vi "Set Master Info.vi"(8 "error in (no error)":errorcluster, 9 "Master #":u32, 10 "Master Name":string, 11 "Item Ref in":T1 format="%.0x") -> (0 "error out":errorcluster, 3 "Item Ref out":T1 format="%.0x")   [LabVIEW 2016, in "Scan Engine Custom Device.lvlib"]
uses:
  Scan Engine Custom Device.lvlib
  <vilib>/NI Veristand/Custom Device API/Custom Device Item Ref.ctl
  Globals/Property Strings.vi
  <vilib>/NI Veristand/Custom Device API/Set Item Property (U32).vi
  <vilib>/NI Veristand/Custom Device API/Custom Device API.lvlib
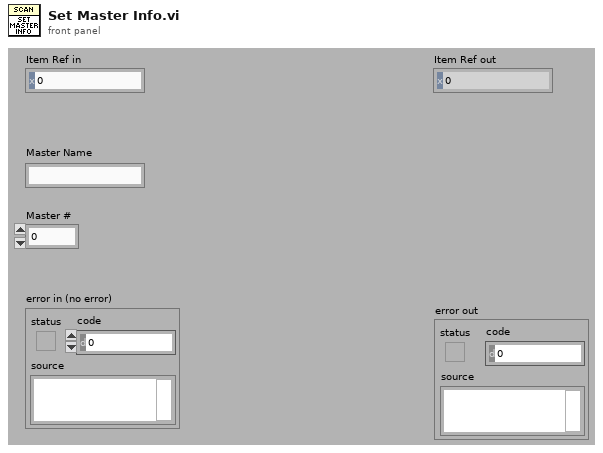
[diagram p1: front panel]
types:
  T1 = typedef "Custom Device API.lvlib/Custom Device Item Ref.ctl" = u64
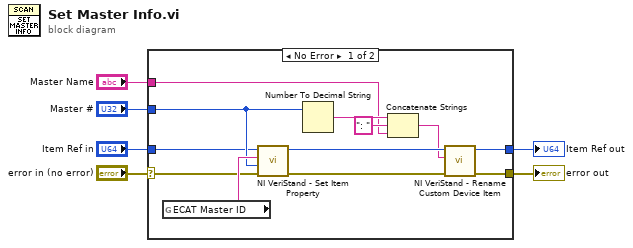
[diagram p0: block diagram]
diagram:
  n1 = case shown="No Error" "error in (no error)" {
    selector: "error in (no error)" -> [w9 w19]
    tunnel: "Item Ref in" -> [w10 w20]
    tunnel: "Master Name" -> [w12 _]
    tunnel: "Master #" -> [w11 _]
    tunnel: [w8 w19] -> w2
    tunnel: [w7 w20] -> w1
    frame No Error {
      n2 = global read "Property Strings.vi" "ECAT Master ID"() -> (w18:string)
      n3 = call-poly <vilib>:"NI VeriStand - Set Item Property.vi"("error in (no error)"=w9, "Value"=w11, "Property Name"=w18, "Item Ref in"=w10) -> ("error out"=w17:errorcluster, "Item Ref out"=w16:T1)  [unwired: 5 in, 1 out]
      n4 = Number To Decimal String(number=w11) -> (decimal integer string=w14:string)  [unwired: 1 in]
      n5 = Concatenate Strings(w14, ": " ("string"), w12) -> (w15:string)
      n6 = call <vilib>:"NI VeriStand - Rename Custom Device Item.vi"("error in (no error)"=w17, "New Name"=w15, "Item Ref in"=w16) -> ("error out"=w8:errorcluster, "Item Ref out"=w7:T1)  [unwired: 1 in, 6 out]
    }
    frame Error {
    }
  }
  "error out" <- w2
  "Item Ref out" <- w1
